vi "Error Code to Error Cluster.vi"(1 "Error Code":i32) -> (0 "Error Out":errorcluster)   [LabVIEW 2019]
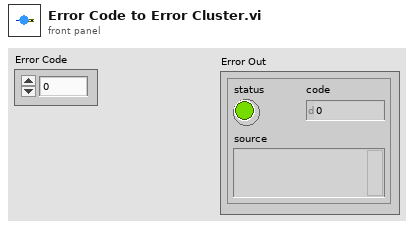
[diagram p1: front panel]
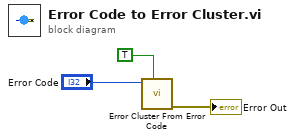
[diagram p0: block diagram]
diagram:
  n1 = call <vilib>:"Error Cluster From Error Code.vi"("show call chain? (False)"=TRUE, "error code (0)"="Error Code") -> ("error out"=→"Error Out":errorcluster)  [unwired: 7 in]
